vi "get_params.vi"(8 "error in (no error)":errorcluster caption="entrée d'erreur (pas d'erreur)", 11 "MLPClassifier.lvclass 2":refnum<class "MLPClassifier.lvclass">) -> (0 "error out":errorcluster caption="sortie d'erreur", 3 "MLPClassifier.lvclass":refnum<class "MLPClassifier.lvclass">)   [LabVIEW 2020, in "MLPClassifier.lvclass"]
uses:
  MLPClassifier.lvclass
  MLPClassifier.lvclass/MLPClassifier.ctl
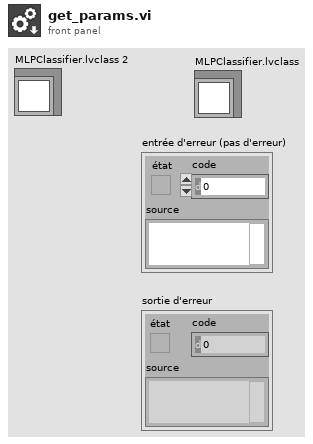
[diagram p1: front panel]
types:
  T1 = typedef "mlp_classifier_params.ctl" = cluster{"hidden_layer_sizes":dbl[], "activation":string, "solver":string, "alpha":dbl, "batch_size":cluster{"batch_size_type":string, "batch_size_int":dbl}, "learning_rate":string, "learning_rate_init":dbl, "power_t":dbl, "max_iter":dbl, "shuffle":bool, "random_state":dbl, "tol":dbl, "verbose":bool, "warm_start":bool, "momentum":dbl, "nesterovs_momentum":bool, "early_stopping":bool, "validation_fraction":dbl, "beta_1":dbl, "beta_2":dbl, "epsilon":dbl, "n_iter_no_change":dbl, "max_fun":dbl}
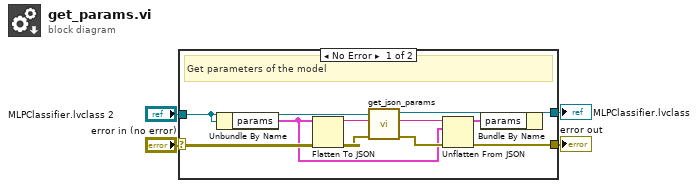
[diagram p0: block diagram]
diagram:
  n1 = case shown="No Error" "error in (no error)" {
    selector: "error in (no error)" -> [w13 w16]
    tunnel: [w5 w16] -> w3
    tunnel: "MLPClassifier.lvclass 2" -> [w10 w17]
    tunnel: [w7 w17] -> w1
    frame No Error {
      # "Get parameters of the model"
      n2 = Unbundle By Name(w10) -> ("params"=w9:T1)
      n3 = Flatten To JSON(anything=w9, error in (no error)=w13) -> (JSON string=w12:string, 11:w11:errorcluster)  [unwired: 1 in]
      n4 = call-dynamic "get_json_params.vi"("error in (no error)"=w11, "format"=w12, "Model en entrée"=w10) -> ("error out"=w14:errorcluster, "valeur renvoyée"=w15:string, "Model en sortie"=w8:refnum<class "MLPClassifier.lvclass">)  [unwired: 6 in]
      n5 = Unflatten From JSON(JSON string=w15, type and defaults=w9, error in (no error)=w14) -> (value=w6:T1, error out=w5:errorcluster)  [unwired: 4 in]
      n6 = Bundle By Name(cluster=w8, "params"=w6) -> (w7:refnum<class "MLPClassifier.lvclass">)
    }
    frame Error {
    }
  }
  "error out" <- w3
  "MLPClassifier.lvclass" <- w1
